vi "Constructor.vi"(8 "error in (no error)":errorcluster, 11 "PPT Path":path) -> (0 "error out":errorcluster, 3 "Parse Presentation out":refnum<class "Parse Presentation.lvclass">)   [LabVIEW 2015, in "Parse Presentation.lvclass"]
uses:
  Parse Presentation.lvclass
  Parse Presentation.lvclass/Parse Presentation.ctl
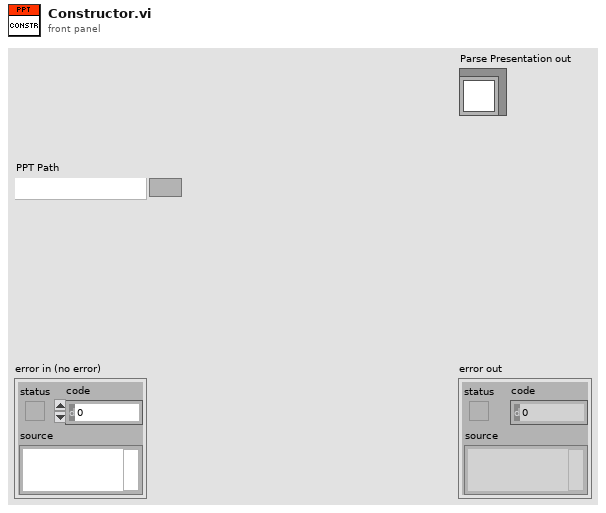
[diagram p1: front panel]
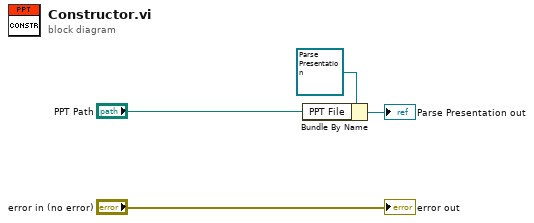
[diagram p0: block diagram]
diagram:
  n1 = Bundle By Name(cluster=refnum<class "Parse Presentation.lvclass"> refnum ("Parse Presentation.lvclass"), "PPT File"="PPT Path") -> (→"Parse Presentation out":refnum<class "Parse Presentation.lvclass">)
  "error out" <- "error in (no error)"
